vi "Team Stats.vi"(11 "Team":refnum<class "Team.lvclass">) -> (2 "Team Stats":T1)   [LabVIEW 2020, in "SquareBattle.lvlib" / "Team.lvclass"]
uses:
  Team.lvclass
  Team Stats.ctl
  Team.lvclass/Team.ctl
  SquareBattle.lvlib
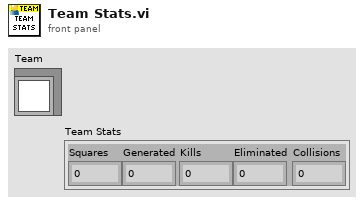
[diagram p1: front panel]
types:
  T1 = typedef "SquareBattle.lvlib/Team Stats.ctl" = cluster{"Squares":i32, "Generated":i32, "Kills":i32, "Eliminated":i32, "Collisions":i32}
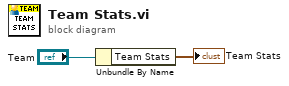
[diagram p0: block diagram]
diagram:
  n1 = Unbundle By Name("Team") -> ("Team Stats"=→"Team Stats":T1)
